vi "Actor Main Run Messages Input Name.vi"() -> (0 "Actor Main Run Messages Terminal Name":string)   [LabVIEW 2018, in "Scripting.lvlib"]
uses:
  Scripting.lvlib
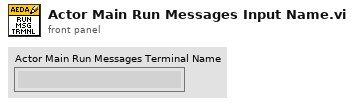
[diagram p1: front panel]
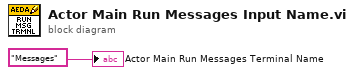
[diagram p0: block diagram]
diagram:
  "Actor Main Run Messages Terminal Name" <- "Messages" ("y")
